vi "Deploy.vi"(8 "error in (no error)":errorcluster, 9 "Name of target":string, 10 "Name of build specification (if empty: deploy all)":string, 11 "Path to project":path) -> (0 "error out":errorcluster)   [LabVIEW 2020, in "NI_App_Builder_API.lvlib"]
doc: "Deploys the output of a build specification to a target. To use this VI, build the build specification using the Build VI."
uses:
  <vilib>/AppBuilder/AB_API_Simple/NI_App_Builder_API.lvlib
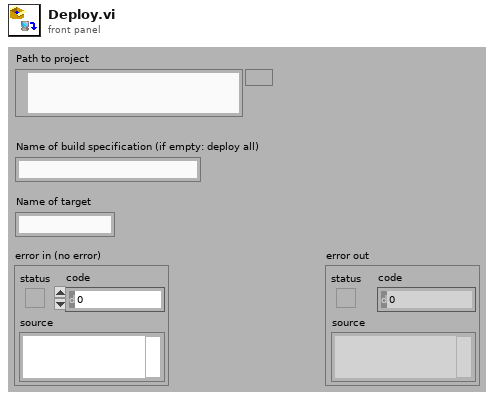
[diagram p1: front panel]
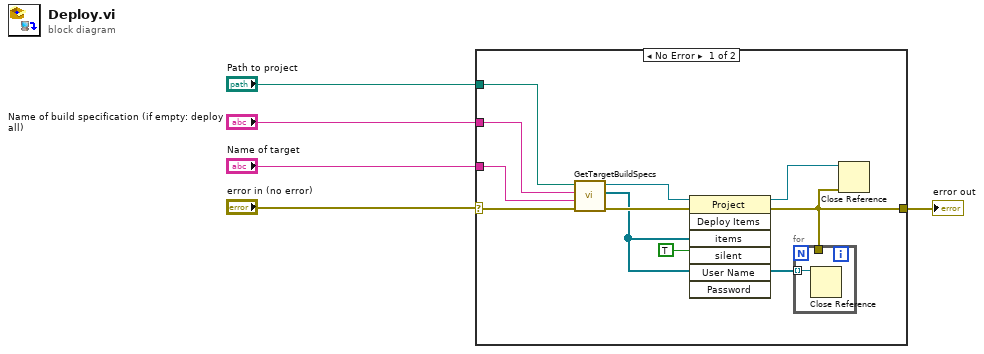
[diagram p0: block diagram]
diagram:
  n1 = case shown="No Error" "error in (no error)" {
    selector: "error in (no error)" -> [w10 w17]
    tunnel: "Path to project" -> [w9 _]
    tunnel: "Name of target" -> [w8 _]
    tunnel: "Name of build specification (if empty: deploy all)" -> [w7 _]
    tunnel: [w15 w17] -> w2
    frame No Error {
      n2 = call <vilib>:"GetTargetBuildSpecs.vi"("error in (no error)"=w10, "Name of target (My Computer)"=w8, "Name of build specification (if empty: get all)"=w7, "Path to project"=w9) -> ("error out"=w12:errorcluster, "buildspec refs"=w11:refnum<vi>[], "project ref"=w13:refnum<vi>)  [unwired: 5 out]
      n3 = invoke class="Project" method="Deploy Items"(reference=w13, error in=w12, "items"=w11, "silent"=TRUE ("Silent")) -> (reference out=w6:refnum<vi>, error out=w15:errorcluster)  [unwired: 3 in, 5 out]
      n4 = for {
        tunnel: w11 -> [w16] mode=indexing
        tunnel: w15 -> [_]
        n5 = Close Reference(reference=w16) -> ()  [unwired: 1 in, 1 out]
      }
      n6 = Close Reference(reference=w6, error in (no error)=w15) -> ()  [unwired: 1 out]
    }
    frame Error {
    }
  }
  "error out" <- w2
